vi "Clear Composite Limit Test.vi"(7 "Enable Auto Clear (T: Enable)":bool=TRUE, 8 "error in (no error)":errorcluster, 9 "Auto Clear Delay Time (0.0001 s)":dbl=0.0001, 10 "Channel (1: Channel 1)":i32(ring)=1 items=["Channel 1"=1, "Channel 2"=2], 11 "VISA resource name":refnum<visa-resource-name>) -> (0 "error out":errorcluster, 3 "VISA resource name out":refnum<visa-resource-name>)   [LabVIEW 2012, in "Keysight B2980 Series.lvlib"]
doc: "Clears the composite limit test results and ports (GPIO lines).\n\n<b>Note(s):</b>\nUse this VI only with other low-level VIs. The high-level VIs automatically incorporate this functionality. This VI does not check the instrument status."
uses:
  Keysight B2980 Series.lvlib
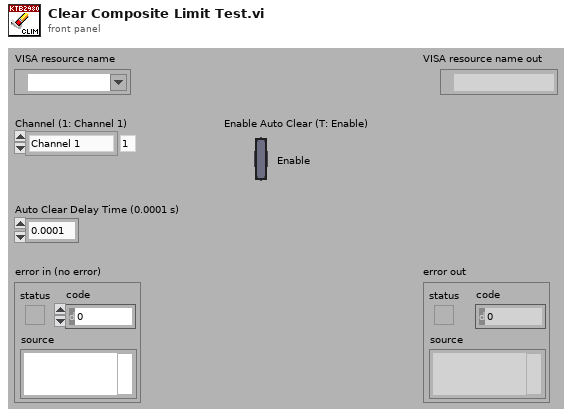
[diagram p1: front panel]
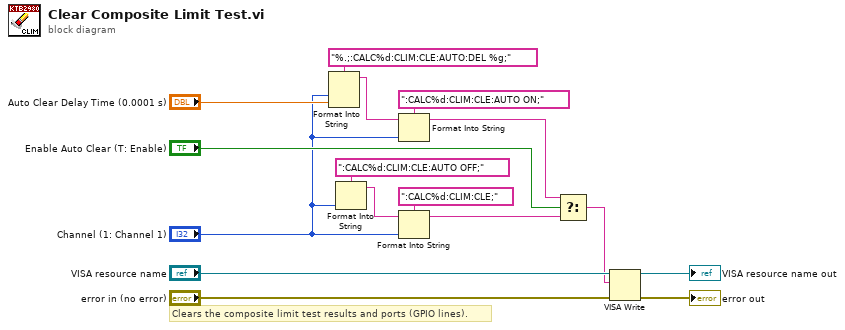
[diagram p0: block diagram]
diagram:
  # "Clears the composite limit test results and ports (GPIO lines)."
  n1 = Format Into String(format string="%.;:CALC%d:CLIM:CLE:AUTO:DEL %g;", "Channel (1: Channel 1)", "Auto Clear Delay Time (0.0001 s)") -> (resulting string=w9:string)  [unwired: 2 in, 1 out]
  n2 = Format Into String(format string=":CALC%d:CLIM:CLE:AUTO OFF;", "Channel (1: Channel 1)") -> (resulting string=w6:string)  [unwired: 2 in, 1 out]
  n3 = Format Into String(format string=":CALC%d:CLIM:CLE:AUTO ON;", initial string=w9, "Channel (1: Channel 1)") -> (resulting string=w8:string)  [unwired: 1 in, 1 out]
  n4 = Format Into String(format string=":CALC%d:CLIM:CLE;", initial string=w6, "Channel (1: Channel 1)") -> (resulting string=w4:string)  [unwired: 1 in, 1 out]
  n5 = Select(t=w8, s="Enable Auto Clear (T: Enable)", f=w4) -> (s? t:f=w3:string)
  n6 = VISA Write(VISA resource name="VISA resource name", write buffer=w3, error in (no error)="error in (no error)") -> (VISA resource name out=→"VISA resource name out":refnum<visa-resource-name>, error out=→"error out":errorcluster)  [unwired: 1 out]
